vi "Plot Helper.vi"   [LabVIEW 2017, in "3D Ribbon Datatype.lvclass"]
doc: "Generates a plot of parallel lines. Multiple references to this VI generate multiple plots for the same graph."
uses:
  <vilib>/Math Plots/3D Math Plots/3D Ribbon/3D Ribbon Datatype/3D Ribbon Datatype.lvclass
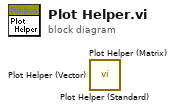
[diagram p0: block diagram]
diagram:
  n1 = call <vilib>:"Plot Helper (Standard).vi"() -> ()  [unwired: 10 in, 2 out]
  n2 = call <vilib>:"Plot Helper (Matrix).vi"() -> ()  [unwired: 10 in, 2 out]
  n3 = call <vilib>:"Plot Helper (Vector).vi"() -> ()  [unwired: 10 in, 2 out]
